vi "Do.vi"(8 "error in (no error)":errorcluster, 10 "Actor in":refnum<class "Actor.lvclass">, 11 "Enqueue Logs Element Msg":refnum<class "Enqueue Logs Element Msg.lvclass">) -> (0 "error out":errorcluster, 2 "Actor out":refnum<class "Actor.lvclass">)   [LabVIEW 2019, in "ErrorLog.lvlib" / "Enqueue Logs Element Msg.lvclass"]
doc: "This VI delivers the message to the actor by calling the appropriate method(s) on the actor."
uses:
  Enqueue Logs Element Msg.lvclass
  <vilib>/ActorFramework/Actor/Actor.lvclass
  ErrorLog/ErrorLog.lvclass
  C:/Program Files (x86)/National Instruments/LabVIEW 2019/vi.lib/ActorFramework/Actor/Actor.lvclass
  Enqueue Logs Element Msg.lvclass/Enqueue Logs Element Msg.ctl
  LogsAbstract/LogsAbstract.lvclass
  Obtain and Save Msg/Obtain and Save Msg.lvclass
  Classes/Error/Error.lvclass
  Modules/ModuleAbstract/ModuleAbstract.lvclass
  C:/Projekty/_Wewnetrzne/PC_ActorFramework/07_Program/LABVIEW/02_Source/SubModules/LogsAbstract/LogsAbstract.lvclass
  C:/Projekty/_Wewnetrzne/PC_ActorFramework/07_Program/LABVIEW/02_Source/Modules/ModuleAbstract/ModuleAbstract.lvclass
  C:/Program Files (x86)/National Instruments/LabVIEW 2019/vi.lib/MGI/Monitored Actor/Monitored Actor/Monitored Actor/Monitored Actor.lvclass
  C:/Projekty/_Wewnetrzne/PC_ActorFramework/07_Program/LABVIEW/02_Source/Classes/EventsAbstract/EventsAbstract.lvclass
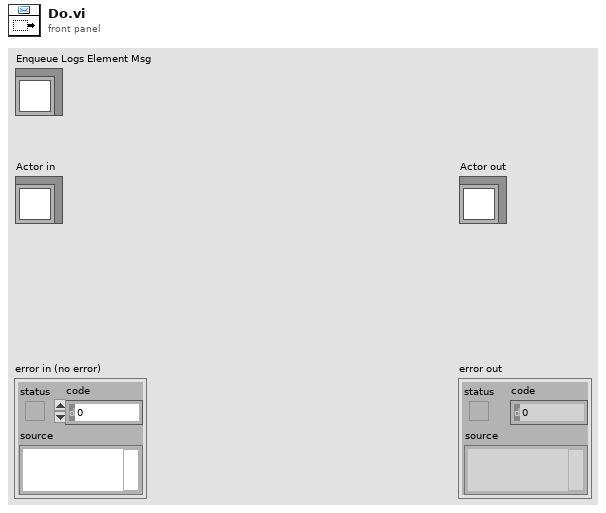
[diagram p1: front panel]
types:
  T1 = typedef "ActorRefContainer.lvlib/ActorRefContainer.lvclass/Active Logs REF.ctl" = cluster{"EventLog":cluster{"ModRef":refnum<class "Message Enqueuer.lvclass">, "UIRef":refnum<class "Message Enqueuer.lvclass">}, "ErrorLog":cluster{"ModRef":refnum<class "Message Enqueuer.lvclass">, "UIRef":refnum<class "Message Enqueuer.lvclass">}}
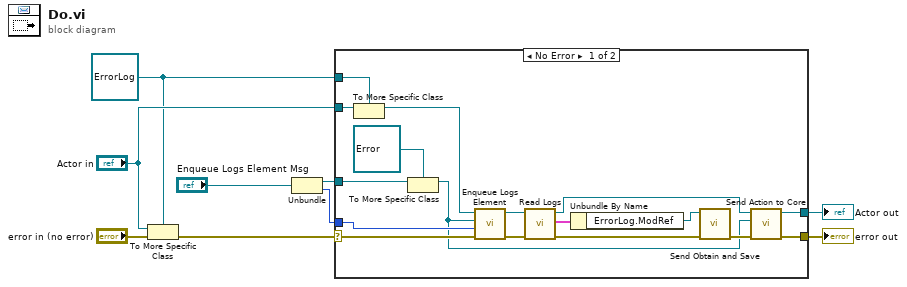
[diagram p0: block diagram]
diagram:
  w3 = refnum<class "ErrorLog.lvclass"> refnum ("Actor in")
  n1 = To More Specific Class(target class=w3, reference="Actor in", error in="error in (no error)") -> (error out=w7:errorcluster)  [unwired: 1 out]
  n2 = Unbundle("Enqueue Logs Element Msg") -> (w2:refnum<class "EventsAbstract.lvclass">, w1:i32)
  n3 = case shown="No Error" w7 {
    selector: w7 -> [w26 w28]
    tunnel: [w21 w28] -> w6
    tunnel: [w10 w27] -> w5
    tunnel: "Actor in" -> [w25 w27]
    tunnel: w3 -> [w24 _]
    tunnel: w2 -> [w18 _]
    tunnel: w1 -> [w22 _]
    frame No Error {
      n4 = To More Specific Class(target class=w24, reference=w25) -> (specific class reference=w23:refnum<class "ErrorLog.lvclass">)  [unwired: 1 in, 1 out]
      n5 = To More Specific Class(target class=refnum<class "Error.lvclass"> refnum ("Error.lvclass"), reference=w18) -> (specific class reference=w17:refnum<class "Error.lvclass">)  [unwired: 1 in, 1 out]
      n6 = call-dynamic "Enqueue Logs Element.vi"("Error In"=w26, "Timeout"=w22, "Event Occured"=w17, "EventLog in"=w23) -> ("Error Out"=w16:errorcluster, "EventLog out"=w14:refnum<class "ErrorLog.lvclass">)  [unwired: 5 in, 1 out]
      n7 = call "Read Logs.vi"("error in (no error)"=w16, "ModuleAbstract in"=w14) -> ("error out"=w15:errorcluster, "Logs"=w13:T1, "ModuleAbstract out"=w11:refnum<class "ErrorLog.lvclass">)  [unwired: 7 in]
      n8 = Unbundle By Name(w13) -> ("ErrorLog.ModRef"=w12:refnum<class "Message Enqueuer.lvclass">)
      n9 = call "Send Obtain and Save.vi"("error in (no error)"=w15, "Message Enqueuer"=w12) -> ("error out"=w20:errorcluster)  [unwired: 8 in, 1 out]
      n10 = call "Send Action to Core.vi"("error in (no error)"=w20, "AnyEvents"=w17, "LogsAbstract in"=w11) -> ("error out"=w21:errorcluster, "LogsAbstract out"=w10:refnum<class "ErrorLog.lvclass">)  [unwired: 7 in]
    }
    frame Error {
      # "If type check fails, pass the original object out again."
    }
  }
  "error out" <- w6
  "Actor out" <- w5
